vi "Create Directory Structure.vi"(8 "error in(no error)":errorcluster, 11 "Dir Path In":path) -> (0 "error out":errorcluster, 3 "Dir Path Out":path)   [LabVIEW 2018]
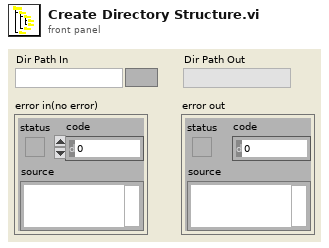
[diagram p1: front panel]
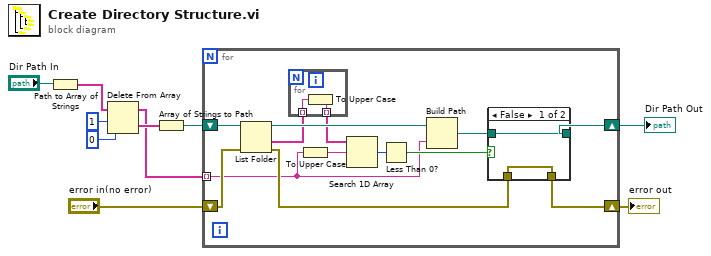
[diagram p0: block diagram]
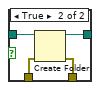
[diagram p2: hidden frame]
diagram:
  n1 = Path to Array of Strings(0:"Dir Path In") -> (2:w9:string[])  [unwired: 1 out]
  n2 = Delete From Array(array=w9, length=1, index=0) -> (deleted portion=w6:string[], array with subset deleted=w4:string[])
  n3 = Array of Strings to Path(0:w6) -> (2:w5:path)  [unwired: 1 in]
  n4 = for {
    shift-right: [w19] -> w3
    shift-left: w5 -> [w22]
    tunnel: w4 -> [w12] mode=indexing
    shift-right: [w15] -> w1
    shift-left: "error in(no error)" -> [w17]
    n5 = List Folder(path=w22, error in=w17) -> (path out=w21:path, folder names=w14:string[], error out=w16:errorcluster)  [unwired: 2 in, 1 out]
    n6 = for {
      tunnel: w14 -> [w25] mode=indexing
      tunnel: [w24] -> w13 mode=indexing
      n7 = To Upper Case(1:w25) -> (0:w24:string)
    }
    n8 = To Upper Case(1:w12) -> (0:w11:string)
    n9 = Search 1D Array(1D array=w13, element=w11) -> (index of element=w23:i32)  [unwired: 1 in]
    n10 = Less Than 0?(x=w23) -> (x < 0?=w18:bool)
    n11 = Build Path(base path=w21, name or relative path=w12) -> (appended path=w20:path)
    n12 = case shown="False" w18 {
      tunnel: w20 -> [w27 w31]
      tunnel: [w27 w30] -> w19
      tunnel: w16 -> [w26 w29]
      tunnel: [w26 w28] -> w15
      frame False {
      }
      frame True {
        n13 = Create Folder(path (use dialog)=w31, error in=w29) -> (created path=w30:path, error out=w28:errorcluster)  [unwired: 1 in, 1 out]
      }
    }
  }
  "Dir Path Out" <- w3
  "error out" <- w1
